vi "Main.vi"() -> ()   [LabVIEW 2016]
uses:
  <vilib>/myRIO/Instrument Drivers/Utilities/Utilities.lvlib
  <vilib>/myRIO/Instrument Drivers/Onboard IO/I2C/I2C.lvlib
  <vilib>/myRIO/Instrument Drivers/Onboard IO/I2C/typedefs/I2C Transfer Rate.ctl
  <vilib>/myRIO/Instrument Drivers/Onboard IO/I2C/typedefs/I2C User Configuration.ctl
  <vilib>/myRIO/Instrument Drivers/Onboard IO/DIO/DIO.lvlib
  <vilib>/platform/TimedLoop/XDataNode/XDataNode.xnode
  <vilib>/Platform/TimedLoop/XDataNode/nitl_modes.ctl
  <vilib>/Platform/TimedLoop/XDataNode/XDNodeRunTimeDep.lvlib
  <vilib>/Platform/TimedLoop/XDataNode/wakeup.ctl
  <vilib>/Platform/TimedLoop/XDataNode/timing_clust.ctl
  <vilib>/Analysis/Matrix/Datatypes/RealMatrix.ctl
  <vilib>/Analysis/Matrix/NI_Matrix.lvlib
panel:
  out "Pitch Angle in degrees":dbl(graph)=-1.8293611669128778
  out "G Matrix":T1=[[0.0001, -5e-09], [0.0, 0.0001]]
  out "F  Matrix":T1=[[1.0, -0.0001], [0.0, 1.0]]
  out "Q'=GQG' (Q scalar =1)":T1=[[1.0000000025e-08, -5e-13], [-5e-13, 1e-08]]
  in  "Kalman Filter = switch off\naccelerometer angle = on":bool=TRUE
  out "H Matrix":T1=[[0.0, 1.0], [1.0, 0.0]]
  out "Angular Velocity for Pitch":dbl(graph)=-0.5
  out "Steady State Kalman Predictor Gain matrixx":T1=[[-7.62521027355318e-05, 0.01032332398776421], [0.031126923690244213, -7.313941036650737e-06]]
  out "Pitch in Degrees":cluster{"t":dbl[], "t":dbl[]}(graph)={"t"=[-97.95005260617272, -96.95056227345667, -95.95107194074062, -94.95158160802457, -93.95209127530853, -92.95260094259248, -91.95311060987643, -90.95362027716038, -89.95412994444433, -88.95463961172828, -87.95514927901223, -86.95565894629618, -85.95616861358015, -84.9566782808641, -83.95718794814805, -82.957697615432, -81.95820728271595, -80.9587169499999, -79.95922661728385, -78.95973628456781, -77.96024595185176, -76.96075561913571, -75.96126528641966, -74.96177495370361, -73.96228462098756, -72.96279428827151, -71.96330395555546, -70.96381362283942, -69.96432329012337, -68.96483295740732, -67.96534262469127, -66.96585229197522, -65.96636195925917, -64.96687162654312, -63.96738129382708, -62.96789096111103, -61.96840062839499, -60.96891029567894, -59.96941996296289, -58.96992963024684, -57.970439297530795, -56.970948964814745, -55.971458632098695, -54.971968299382645, -53.9724779666666, -52.97298763395055, -51.9734973012345, -50.97400696851845, -49.97451663580241, -48.97502630308636, -47.97553597037031, -46.976045637654266, -45.976555304938216, -44.977064972222166, -43.977574639506116, -42.97808430679007, -41.97859397407402, -40.97910364135797, -39.97961330864192, -38.98012297592588, -37.98063264320983, -36.98114231049378, -35.98165197777773, -34.98216164506169, -33.98267131234564, -32.98318097962959, -31.98369064691354, -30.984200314197494, -29.984709981481444, -28.985219648765398, -27.985729316049348, -26.9862389833333, -25.98674865061725, -24.987258317901205, -23.987767985185155, -22.988277652469108, -21.988787319753058, -20.98929698703701, -19.98980665432096, -18.990316321604915, -17.990825988888865, -16.99133565617282, -15.99184532345677, -14.992354990740722, -13.992864658024674, -12.993374325308626, -11.993883992592577, -10.994393659876529, -9.99490332716048, -8.995412994444433, -7.995922661728385, -6.996432329012337, -5.996941996296289, -4.99745166358024, -3.9979613308641926, -2.9984709981481443, -1.9989806654320963, -0.9994903327160481, 0.0, 0.9994903327160481, 1.9989806654320963, 2.9984709981481443, 3.9979613308641926, 4.99745166358024, 5.996941996296289, 6.996432329012337, 7.995922661728385, 8.995412994444433, 9.99490332716048, 10.994393659876529, 11.993883992592577, 12.993374325308626, 13.992864658024674, 14.992354990740722, 15.99184532345677, 16.99133565617282, 17.990825988888865, 18.990316321604915, 19.98980665432096, 20.98929698703701, 21.988787319753058, 22.988277652469108, 23.987767985185155, 24.987258317901205, 25.98674865061725, 26.9862389833333, 27.985729316049348, 28.985219648765398, 29.984709981481444, 30.984200314197494, 31.98369064691354, 32.98318097962959, 33.98267131234564, 34.98216164506169, 35.98165197777773, 36.98114231049378, 37.98063264320983, 38.98012297592588, 39.97961330864192, 40.97910364135797, 41.97859397407402, 42.97808430679007, 43.977574639506116, 44.977064972222166, 45.976555304938216, 46.976045637654266, 47.97553597037031, 48.97502630308636, 49.97451663580241, 50.97400696851845, 51.9734973012345, 52.97298763395055, 53.9724779666666, 54.971968299382645, 55.971458632098695, 56.970948964814745, 57.970439297530795, 58.96992963024684, 59.96941996296289, 60.96891029567894, 61.96840062839499, 62.96789096111103, 63.96738129382708, 64.96687162654312, 65.96636195925917, 66.96585229197522, 67.96534262469127, 68.96483295740732, 69.96432329012337, 70.96381362283942, 71.96330395555546, 72.96279428827151, 73.96228462098756, 74.96177495370361, 75.96126528641966, 76.96075561913571, 77.96024595185176, 78.95973628456781, 79.95922661728385, 80.9587169499999, 81.95820728271595, 82.957697615432, 83.95718794814805, 84.9566782808641, 85.95616861358015, 86.95565894629618, 87.95514927901223, 88.95463961172828, 89.95412994444433, 90.95362027716038, 91.95311060987643, 92.95260094259248, 93.95209127530853, 94.95158160802457, 95.95107194074062, 96.95056227345667, 97.95005260617272, 98.94954293888877, 99.94903327160482], "t"=[3.1284492081536053, 3.096526257049997, 3.064603305946389, 3.0326803548427805, 3.0007574037391724, 2.9688344526355643, 2.936911501531956, 2.9049885504283477, 2.8730655993247396, 2.8411426482211315, 2.809219697117523, 2.777296746013915, 2.7453737949103068, 2.7134508438066987, 2.68152789270309, 2.649604941599482, 2.617681990495874, 2.585759039392266, 2.5538360882886573, 2.521913137185049, 2.489990186081441, 2.4580672349778325, 2.4261442838742244, 2.3942213327706163, 2.3622983816670082, 2.3303754305633997, 2.2984524794597916, 2.2665295283561835, 2.2346065772525754, 2.202683626148967, 2.1707606750453587, 2.1388377239417506, 2.1069147728381425, 2.074991821734534, 2.043068870630926, 2.011145919527318, 1.9792229684237095, 1.9473000173201012, 1.915377066216493, 1.8834541151128847, 1.8515311640092766, 1.8196082129056683, 1.7876852618020602, 1.755762310698452, 1.7238393595948438, 1.6919164084912355, 1.6599934573876274, 1.628070506284019, 1.596147555180411, 1.5642246040768026, 1.5323016529731945, 1.5003787018695862, 1.468455750765978, 1.4365327996623698, 1.4046098485587615, 1.3726868974551534, 1.340763946351545, 1.308840995247937, 1.2769180441443286, 1.2449950930407205, 1.2130721419371122, 1.1811491908335041, 1.1492262397298958, 1.1173032886262877, 1.0853803375226794, 1.0534573864190713, 1.021534435315463, 0.9896114842118547, 0.9576885331082465, 0.9257655820046383, 0.8938426309010301, 0.8619196797974219, 0.8299967286938137, 0.7980737775902055, 0.7661508264865973, 0.734227875382989, 0.7023049242793807, 0.6703819731757725, 0.6384590220721643, 0.6065360709685561, 0.5746131198649479, 0.5426901687613397, 0.5107672176577315, 0.47884426655412327, 0.44692131545051506, 0.41499836434690685, 0.38307541324329863, 0.35115246213969037, 0.31922951103608216, 0.28730655993247395, 0.25538360882886574, 0.22346065772525753, 0.19153770662164932, 0.15961475551804108, 0.12769180441443287, 0.09576885331082466, 0.06384590220721643, 0.03192295110360822, -0.0, -0.03192295110360822, -0.06384590220721643, -0.09576885331082466, -0.12769180441443287, -0.15961475551804108, -0.19153770662164932, -0.22346065772525753, -0.25538360882886574, -0.28730655993247395, -0.31922951103608216, -0.35115246213969037, -0.38307541324329863, -0.41499836434690685, -0.44692131545051506, -0.47884426655412327, -0.5107672176577315, -0.5426901687613397, -0.5746131198649479, -0.6065360709685561, -0.6384590220721643, -0.6703819731757725, -0.7023049242793807, -0.734227875382989, -0.7661508264865973, -0.7980737775902055, -0.8299967286938137, -0.8619196797974219, -0.8938426309010301, -0.9257655820046383, -0.9576885331082465, -0.9896114842118547, -1.021534435315463, -1.0534573864190713, -1.0853803375226794, -1.1173032886262877, -1.1492262397298958, -1.1811491908335041, -1.2130721419371122, -1.2449950930407205, -1.2769180441443286, -1.308840995247937, -1.340763946351545, -1.3726868974551534, -1.4046098485587615, -1.4365327996623698, -1.468455750765978, -1.5003787018695862, -1.5323016529731945, -1.5642246040768026, -1.596147555180411, -1.628070506284019, -1.6599934573876274, -1.6919164084912355, -1.7238393595948438, -1.755762310698452, -1.7876852618020602, -1.8196082129056683, -1.8515311640092766, -1.8834541151128847, -1.915377066216493, -1.9473000173201012, -1.9792229684237095, -2.011145919527318, -2.043068870630926, -2.074991821734534, -2.1069147728381425, -2.1388377239417506, -2.1707606750453587, -2.202683626148967, -2.2346065772525754, -2.2665295283561835, -2.2984524794597916, -2.3303754305633997, -2.3622983816670082, -2.3942213327706163, -2.4261442838742244, -2.4580672349778325, -2.489990186081441, -2.521913137185049, -2.5538360882886573, -2.585759039392266, -2.617681990495874, -2.649604941599482, -2.68152789270309, -2.7134508438066987, -2.7453737949103068, -2.777296746013915, -2.809219697117523, -2.8411426482211315, -2.8730655993247396, -2.9049885504283477, -2.936911501531956, -2.9688344526355643, -3.0007574037391724, -3.0326803548427805, -3.064603305946389, -3.096526257049997, -3.1284492081536053, -3.1603721592572134, -3.192295110360822]}
  out "Raw accelerometer angle in degrees":dbl=-1.8293611669128778
  out "State Predicted Estimate X^(k+1/k)":dbl[](array[numeric])=[-1.7557452195435928, 0.08364774980311916]
  out "Y Gyro rate":i16=22
  in  "Y offset trim gyro velocity":i16=-244
  out "Rx accel":i16=-384
  in  "X degrees  offset trim angle":dbl=-2.4999999999999982 min=-20.0 max=20.0 step=0.1
  out "X displacement degrees from Kalman filter\nUse this for Segway balance":dbl=-1.7557452195435928 format="%#_5g"
  in  "X offset trim gyro velocity":i16=60
  out "Rz acc":i16=15184
  out "Ry acc":i16=-1150
  out "X Gyro rate":i16=-5
  in  "?":bool
  # "MPU6050 with steady-state\nKalman Filter (Wiener state filter)"
  # "3.3V --> VCC\n\nGND --> dig GND\n\nSDA --> 34\n\nSCL --> 32"
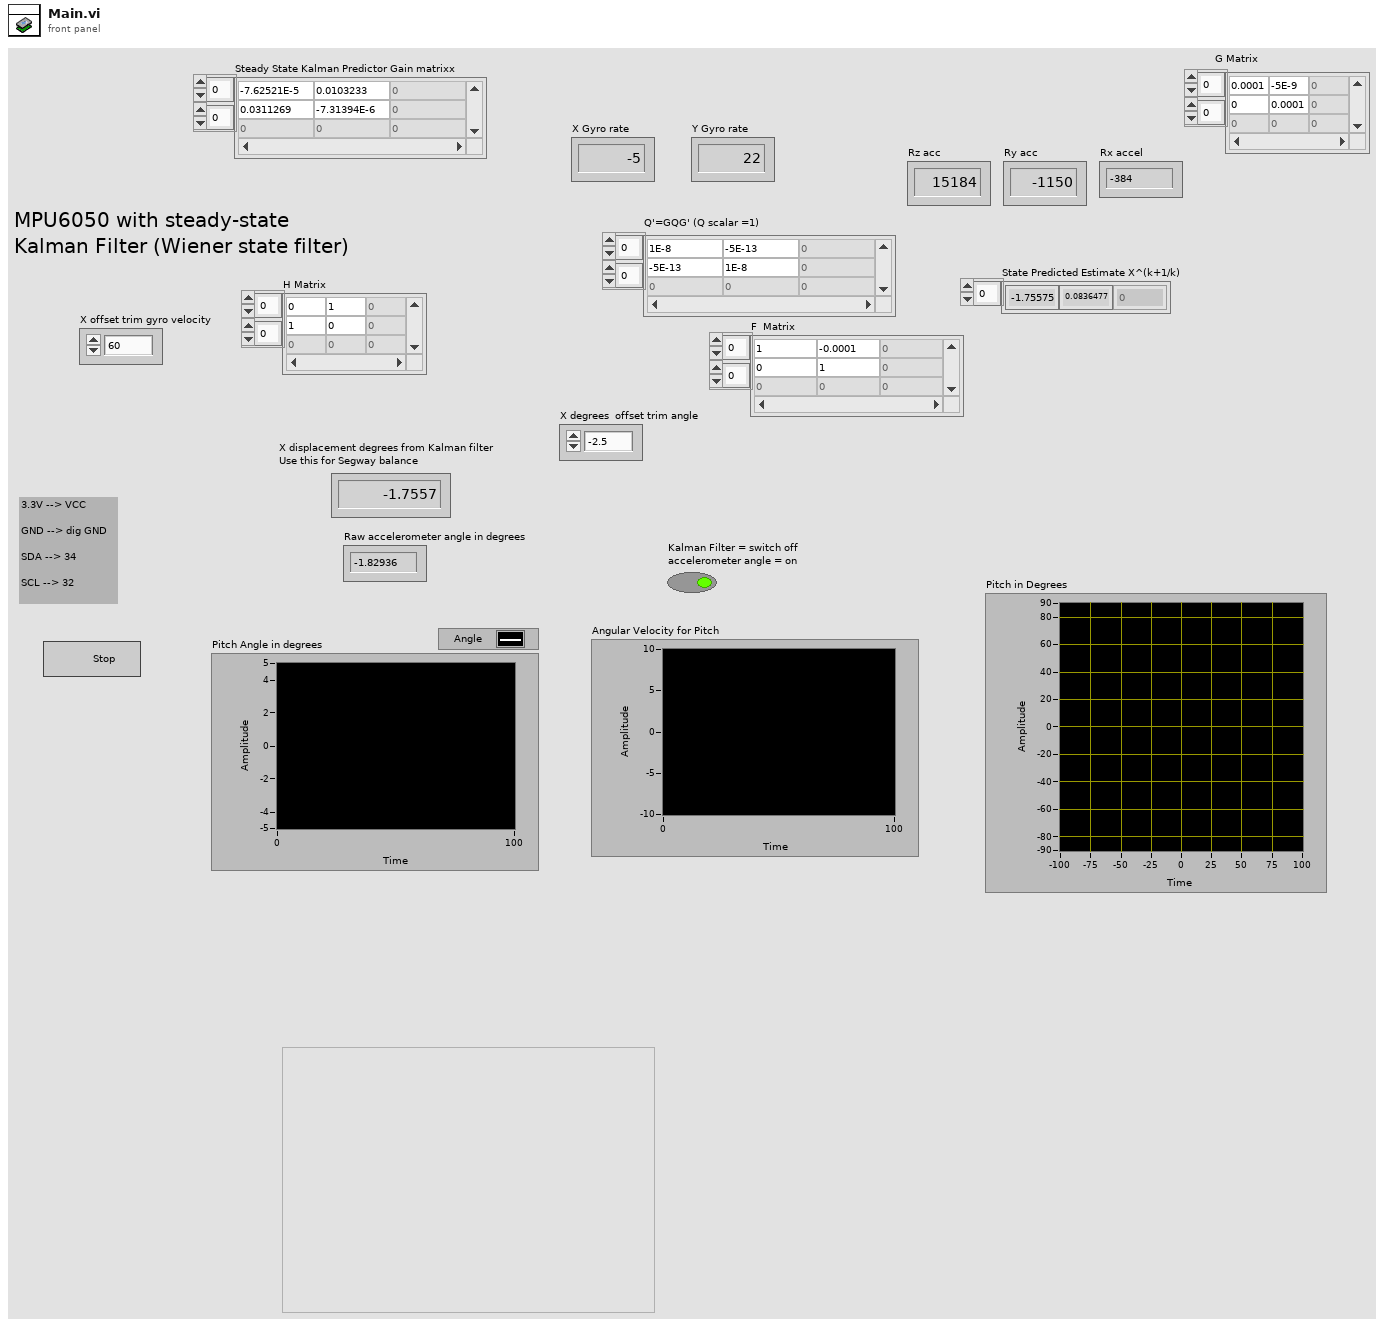
[diagram p1: front panel]
types:
  T1 = typedef "NI_Matrix.lvlib/RealMatrix.ctl" = dbl[][]
  T2 = typedef "I2C.lvlib/I2C User Configuration.ctl" = cluster{"I2C Transfer Rate":T3}
  T3 = typedef "I2C.lvlib/I2C Transfer Rate.ctl" = enum16{"Standard mode (100 kbps)", "Fast mode (400 kbps)"}
  T4 = typedef "I2C.lvlib/I2C Reference.ctl" = cluster{"myRIO Reference":T5, "I2C Channels Enum":T9, "I2C Configuration":T10}
  T5 = typedef "myRIO Generic Hardware Reference.ctl" = cluster{"myRIO Model":T6, "myRIO Hardware Reference":T7}
  T6 = typedef "Hardware Version Enum.ctl" = enum16{"Unknown", "myRIO-1900", "myRIO-1950", "roboRIO", "NI ELVIS RIO CM"}
  T7 = typedef "myRIO v1.0 Reference.ctl" = cluster{"Generic FPGA Reference":T8, "Allow multiple opens":bool}
  T8 = typedef "Generic FPGA Reference.ctl" = refnum<k20>
  T9 = typedef "I2C Channels Enum.ctl" = enum16{"Not Connected", "A/I2C", "B/I2C", "I2C/I2C"}
  T10 = typedef "I2C.lvlib/I2C Configuration.ctl" = cluster{"I2C Transfer Rate":T3}
  T11 = typedef "DIO.lvlib/DIO Reference.ctl" = cluster{"myRIO Reference":T5, "DIO Channels List":T12}
  T12 = typedef "DIO Channels List.ctl" = T13[]
  T13 = typedef "DIO Channels Enum.ctl" = enum16{"Not Connected", "C/DIO0", "C/DIO1", "C/DIO2", "C/DIO3", "C/DIO4", "C/DIO5", "C/DIO6", "C/DIO7", "A/DIO0", "A/DIO1", "A/DIO2", "A/DIO3", "A/DIO4", "A/DIO5", "A/DIO6", "A/DIO7", "A/DIO8", "A/DIO9", "A/DIO10", "A/DIO11", "A/DIO12", "A/DIO13", "A/DIO14", "A/DIO15", "B/DIO0", "B/DIO1", "B/DIO2", "B/DIO3", "B/DIO4", "B/DIO5", "B/DIO6", "B/DIO7", "B/DIO8", "B/DIO9", "B/DIO10", "B/DIO11", "B/DIO12", "B/DIO13", "B/DIO14", "B/DIO15", "LED0", "LED1", "LED2", "LED3", "Button0", "DIO/DIO0", "DIO/DIO1", "DIO/DIO2", "DIO/DIO3", "DIO/DIO4", "DIO/DIO5", "DIO/DIO6", "DIO/DIO7", "DIO/DIO8", "DIO/DIO9", "SPI/CS0", "SPI/CS1", "SPI/CS2", "SPI/CS3", "LED RADIO (Green)", "LED RADIO (Red)", "LED COMM (Green)", "LED COMM (Red)", "LED MODE (Green)", "LED MODE (Red)"}
  T14 = typedef "XDNodeRunTimeDep.lvlib/timing_clust.ctl" = cluster{"Expected End [f-1]":u64, "Actual End [f-1]":u64, "Finished Late? [f-1]":bool, "Expected End [i-1]":u64, "Actual End [i-1]":u64, "Finished Late? [i-1]":bool, "Expected Start [i]":u64, "Actual Start [i]":u64, "Expected Start [f]":u64, "Actual Start [f]":u64, "Source Name":string, "Structure Name":string, "Period":i64, "Deadline":i64, "Offset":i64, "Start":i64, "Priority":i32, "Timeout":i32, "Mode":T15, "Wakeup Reason":T16, "Error":errorcluster, "Source Type":string, "Secondary Source Type":string, "Global End Time":u64, "Global Start Time":u64, "Frame Duration":u64, "Iteration Duration":u64, "Assigned CPU":i32, "I/O Scan Engine Mode":u32}
  T15 = typedef "XDNodeRunTimeDep.lvlib/nitl_modes.ctl" = enum32{"No Change", "Process missed periods, maintain original phase", "Discard missed periods, maintain original phase", "Process missed periods, ignore original phase", "Discard missed periods, ignore original phase"}
  T16 = typedef "XDNodeRunTimeDep.lvlib/wakeup.ctl" = enum32{"Normal", "Aborted", "Asynchronous wakeup", "Timing source error", "Timed loop error", "Timeout"}
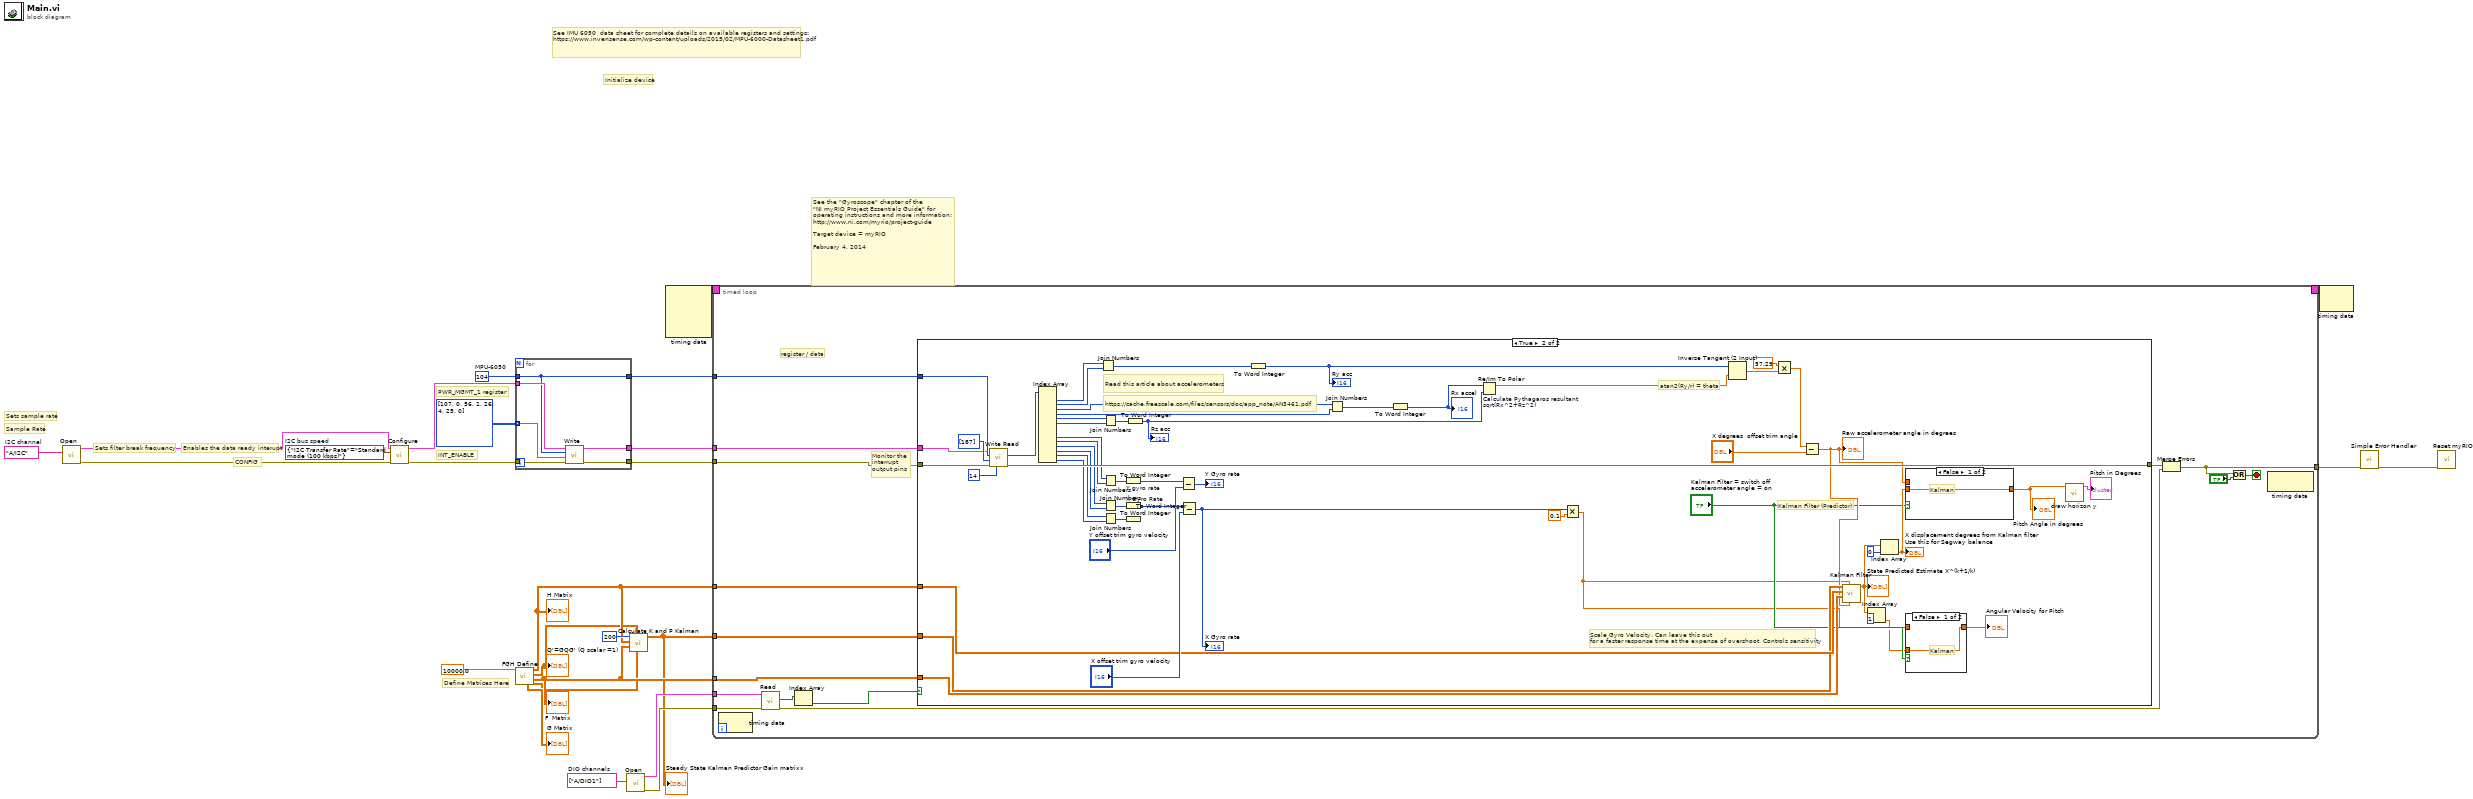
[diagram p0: block diagram]
diagram:
  w13 = tag[] ["A/DIO1"]  # DIO channels
  w24 = T2 {"I2C Transfer Rate"=enum."Standard mode (100 kbps)"}  # I2C bus speed
  w9 = tag "A/I2C"  # I2C channel
  w15 = u8 104  # MPU-6050
  # "Define Matrices Here"
  # "Sets sample rate"
  # "Sample Rate"
  # "Sets filter break frequency"
  # "CONFIG"
  # "INT_ENABLE"
  # "Enables the data ready interupt"
  # "See the \"Gyroscope\" chapter of the\n\"NI myRIO Project Essentials Guide\" for\noperating instructions and more information: \nhttp://www.ni.com/myrio/project-guide\n\nTarget device = myRIO\n\nFebruary 4, 2014"
  # "PWR_MGMT_1 register"
  # "Initialize device"
  # "See IMU 6050  data sheet for complete details on available registers and settings:\nhttps://www.invensense.com/wp-content/uploads/2015/02/MPU-6000-Datasheet1.pdf"
  # "register / data"
  n1 = call <vilib>:"Open.vi"("Channel Name"=w9) -> ("error out"=w22:errorcluster, "I2C Ref Out"=w23:T4)  [unwired: 9 in]
  n2 = call <vilib>:"Configure.vi"("error in (no error)"=w22, "I2C User Configuration"=w24, "I2C Ref In"=w23) -> ("error out"=w16:errorcluster, "I2C Ref Out"=w17:T4)  [unwired: 7 in]
  n3 = for {
    tunnel: [w32] -> w21
    tunnel: [w31] -> w20
    tunnel: [w27] -> w19
    tunnel: u8[][] [[107, 0], [56, 1], [26, 4], [25, 0]] ("Bytes to Write") -> [w30] mode=indexing
    tunnel: w17 -> [w29]
    tunnel: w16 -> [w28]
    tunnel: w15 -> [w27]
    n4 = call <vilib>:"Write.vi"("error in (no error)"=w28, "Bytes to Write"=w30, "Slave Address (7-bit)"=w27, "I2C Ref In"=w29) -> ("error out"=w32:errorcluster, "I2C Ref Out"=w31:T4)  [unwired: 6 in]
  }
  n5 = call "FGH Define.vi"("Sampling Freqauency (Hz)"=10000.0) -> ("G Matrix"=→"G Matrix":T1, "F  Matrix"=w6:T1, "Q = GQG'"=w2:T1, "H Matrix"=w4:T1, "R Matrix"=w5:T1)  [unwired: 6 in]
  "H Matrix" <- w4
  "Q'=GQG' (Q scalar =1)" <- w2
  "F  Matrix" <- w6
  n6 = call <vilib>:"Open.vi"("Channel Names"=w13) -> ("error out"=w14:errorcluster, "DIO Ref Out"=w10:T11)  [unwired: 9 in]
  n7 = call "Calculate K and P Kalman.vi"("R Matrix"=w5, "Q'=GQG' (Q scalar =1)"=w2, "F  Matrix"=w6, "H Matrix"=w4, "Number of iterations"=200) -> ("Steady State Kalman Predictor Gain matrixx"=w3:T1)  [unwired: 4 in, 2 out]
  "Steady State Kalman Predictor Gain matrixx" <- w3
  n8 = node-c288() -> (w12:T14)  [unwired: 4 in]
  n9 = timed-loop {
    tunnel: [w38] -> w25
    tunnel: w19 -> [w43]
    tunnel: w21 -> [w45]
    tunnel: w20 -> [w44]
    tunnel: w14 -> [w42]
    timing: w12 -> [_]
    timing-out: [_] -> w11
    tunnel: w10 -> [w37]
    tunnel: w6 -> [w35]
    tunnel: w4 -> [w34]
    tunnel: w3 -> [w33]
    stop <- w47 stop-if-true
    # "Monitor the\ninterrupt\noutput pins"
    n10 = node-c288() -> ()  [unwired: 1 in, 1 out]
    n11 = call <vilib>:"Read.vi"("error in (no error)"=w42, "DIO Ref In"=w37) -> ("error out"=w36:errorcluster, "Values"=w39:bool[])  [unwired: 7 in, 1 out]
    n12 = Index Array "Index Array"(array=w39) -> (element=w40:bool)  [unwired: 1 in]
    n13 = case shown="True" w40 {
      tunnel: w45 -> [w50 w96]
      tunnel: w44 -> [_ w97]
      tunnel: w43 -> [_ w100]
      tunnel: [w50 w99] -> w41
      tunnel: w35 -> [_ w73]
      tunnel: w34 -> [_ w63]
      tunnel: w33 -> [_ w62]
      frame False {
        # "INT2 (data ready) deasserted"
      }
      frame True {
        # "Kalman Filter (Predictor)"
        # "Scale Gyro Velocity. Can leave this out\nfor a faster response time at the expense of overshoot. Controls sensitivity"
        # "atan2(Ry/r) = theta"
        # "https://cache.freescale.com/files/sensors/doc/app_note/AN3461.pdf"
        # "Read this article about accelerometers"
        n14 = call <vilib>:"Write Read.vi"("Byte Count"=u32 14, "error in (no error)"=w96, "Bytes to Write"=u8[] [187], "Slave Address (7-bit)"=w100, "I2C Ref In"=w97) -> ("error out"=w99:errorcluster, "Bytes Read"=w98:u8[])  [unwired: 3 in, 1 out]
        n15 = Index Array "Index Array"(array=w98) -> (element #1=w95:u8, element #2=w94:u8, element #3=w83:u8, element #4=w82:u8, element #5=w93:u8, element #6=w92:u8, element #9=w79:u8, element #10=w80:u8, element #11=w91:u8, element #12=w90:u8, element #13=w89:u8, element #14=w88:u8)  [unwired: 14 in, 2 out]
        n16 = Join Numbers(hi=w95, lo=w94) -> ((hi.lo)=w104:u16)
        n17 = Join Numbers(hi=w93, lo=w92) -> ((hi.lo)=w103:u16)
        n18 = Join Numbers(hi=w79, lo=w80) -> ((hi.lo)=w78:u16)
        n19 = Join Numbers(hi=w91, lo=w90) -> ((hi.lo)=w87:u16)
        n20 = Join Numbers(hi=w89, lo=w88) -> ((hi.lo)=w86:u16)
        n21 = To Word Integer "Y gyro rate"(number=w78) -> (16bit integer=w77:i16)
        n22 = To Word Integer "X Gyro Rate"(number=w87) -> (16bit integer=w85:i16)
        n23 = To Word Integer(number=w86) -> ()  [unwired: 1 out]
        n24 = To Word Integer(number=w103) -> (16bit integer=w74:i16)
        "Rz acc" <- w74
        n25 = Subtract(x=w77, y="Y offset trim gyro velocity") -> (x-y=→"Y Gyro rate":i16)
        n26 = Subtract(x=w85, y="X offset trim gyro velocity") -> (x-y=w66:i16)
        "X Gyro rate" <- w66
        n27 = To Word Integer(number=w104) -> (16bit integer=w58:i16)
        "Ry acc" <- w58
        n28 = Join Numbers(hi=w83, lo=w82) -> ((hi.lo)=w81:u16)
        n29 = To Word Integer(number=w81) -> (16bit integer=w59:i16)
        "Rx accel" <- w59
        n30 = Re/Im To Polar "Calculate Pythagaros resultant sqrt(Rx^2+Rz^2)"(2:w74, 3:w59) -> (1:w65:dbl)  [unwired: 1 out]
        n31 = Multiply(x=w66, y=0.1) -> (x*y=w51:dbl)
        n32 = Inverse Tangent (2 Input)(1:w65, 2:w58) -> (0:w67:dbl)
        n33 = Multiply(x=57.29, y=w67) -> (x*y=w72:dbl)
        n34 = Subtract(x=w72, y="X degrees  offset trim angle") -> (x-y=w57:dbl)
        "Raw accelerometer angle in degrees" <- w57
        n35 = call "Kalman Filter.vi"("Observations2\naccelerometer angle"=w57, "Observations1\nGyro"=w51, "F  Matrix"=w73, "H Matrix"=w63, "Steady State Kalman Predictor Gain matrixx"=w62) -> ("State Predicted Estimate X^(k+1/k)"=w61:dbl[])  [unwired: 6 in]
        "State Predicted Estimate X^(k+1/k)" <- w61
        n36 = Index Array(array=w61, index=1) -> (element=w52:dbl)
        n37 = Index Array(array=w61, index=0) -> (element=w55:dbl)
        "X displacement degrees from Kalman filter\nUse this for Segway balance" <- w55
        n38 = case shown="False" "Kalman Filter = switch off\naccelerometer angle = on" {
          tunnel: w57 -> [_ w108]
          tunnel: [w107 w108] -> w56
          tunnel: w55 -> [w107 _]
          frame False {
            # "Kalman"
          }
          frame True {
            # "Accelerometer\nangle on its own"
          }
        }
        "Pitch Angle in degrees" <- w56
        n39 = case shown="False" "Kalman Filter = switch off\naccelerometer angle = on" {
          tunnel: w51 -> [_ w106]
          tunnel: [w105 w106] -> w54
          tunnel: w52 -> [w105 _]
          frame False {
            # "Kalman"
          }
          frame True {
          }
        }
        "Angular Velocity for Pitch" <- w54
        n40 = call "draw horizon y.vi"("angle in degrees in"=w56) -> ("x-y graph"=→"Pitch in Degrees":cluster{"t":dbl[], "t":dbl[]})  [unwired: 10 in]
      }
    }
    n41 = Merge Errors "Merge Errors"(w41, w36) -> (w38:errorcluster)
    n42 = Or(x=w38, y="?") -> (x .or. y?=w47:bool)
    n43 = node-c288() -> ()  [unwired: 1 in, 1 out]
  }
  n44 = node-c288(w11) -> ()  [unwired: 1 out]
  n45 = call <vilib>:"Simple Error Handler.vi"("error in (no error)"=w25) -> ("error out"=w26:errorcluster)  [unwired: 4 in, 4 out]
  n46 = call <vilib>:"Reset myRIO.vi"("error in (no error)"=w26) -> ()  [unwired: 10 in, 1 out]
